vi "schedule_triggers.vi"(8 "error in (no error)":errorcluster, 10 "scheduled trigger":T1[](array[typedef]), 11 "DL090503StimulatorScaffold in":refnum<class "StimulatorDL090503Scaffold.lvclass">) -> (0 "error out":errorcluster, 3 "DL090503StimulatorScaffold out":refnum<class "StimulatorDL090503Scaffold.lvclass">)   [LabVIEW 2010, in "StimulatorDL090503Scaffold.lvclass"]
uses:
  StimulatorDL090503Scaffold.lvclass
  schedule_entry_cluster.ctl
  common/classes/GenericToplevelComponent/GenericToplevelComponent/common_trigger_enum.ctl
  StimulatorDL090503Scaffold.lvclass/StimulatorDL090503Scaffold.ctl
  common/classes/GenericToplevelComponent/GenericToplevelComponent/GenericToplevelComponent.lvclass
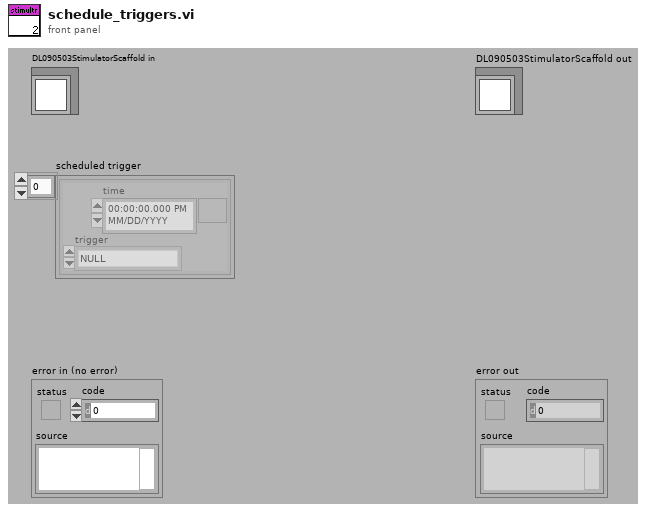
[diagram p1: front panel]
types:
  T1 = typedef "StimulatorDL090503Scaffold.lvclass/schedule_entry_cluster.ctl" = cluster{"time":timestamp, "trigger":T2}
  T2 = typedef "GenericToplevelComponent.lvclass/common_trigger_enum.ctl" = enum16{"NULL", "initialise", "terminate", "fetch command", "fetch data", "attach observer", "register as observer", "detach observer", "acknowledge", "start", "stop", "sweep started", "sweep finished", "experiment started", "experiment stopped"}
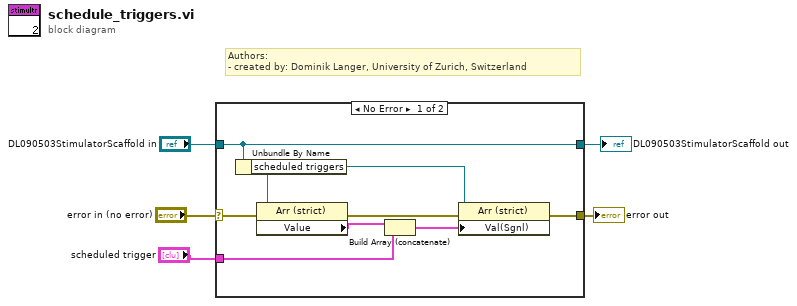
[diagram p0: block diagram]
diagram:
  # "Authors: \n- created by: Dominik Langer, University of Zurich, Switzerland"
  n1 = case shown="No Error" "error in (no error)" {
    selector: "error in (no error)" -> [w12 w15]
    tunnel: [w7 w15] -> w4
    tunnel: [w10 w14] -> w2
    tunnel: "DL090503StimulatorScaffold in" -> [w10 w14]
    tunnel: "scheduled trigger" -> [w13 _]
    frame No Error {
      n2 = Unbundle By Name(w10) -> ("scheduled triggers"=w9:refnum<vi>)
      n3 = property class="Arr (strict)"(reference=w9, error in=w12) -> (error out=w8:errorcluster, "Value"=w11:T1[])  [unwired: 1 out]
      n4 = Build Array (concatenate)(w11, w13) -> (w6:T1[])
      n5 = property class="Arr (strict)"(reference=w9, error in=w8, "Val(Sgnl)"=w6) -> (error out=w7:errorcluster)  [unwired: 1 out]
    }
    frame Error {
    }
  }
  "error out" <- w4
  "DL090503StimulatorScaffold out" <- w2
